vi "BonOMM-SAOMM.vi"() -> ()   [LabVIEW 2019] (continued)
                            n2356 = One Button Dialog(message="Errreur lors du déplacement de la roue") -> ()  [unwired: 1 in, 1 out]
                          }
                          frame True {
                          }
                        }
                      }
                      frame True {
                      }
                    }
                  }
                  frame #3 {
                    w6291 = u8 0 ("byte count")
                    w6301 = FALSE
                    n2357 = local read "Annulation en cours"() -> (w6288:bool)
                    n2358 = case shown="Faux" w6288 {
                      tunnel: w6300 -> [w6323 _]
                      frame False {
                        n2359 = call "MC-BonOMM_talker.vi"("MC-BonOMM VRN"=w6323, "Commande"="q" ("write buffer"), "byte count"=u32 1, "Timeout (ms)"=1000, "answer=command?"=FALSE) -> ("Answer"=w6318:string, "ok ?"=w6317:bool)
                        n2360 = local write "MC_connect"(w6317) -> ()
                        n2361 = Decimal String To Number(string=w6318) -> (number=w6322:i32)  [unwired: 2 in, 1 out]
                        n2362 = local write "F#"(w6322) -> ()
                        n2363 = case shown="1..6" w6322 {
                          selector: w6322 -> [w6333 _]
                          frame 1..6 {
                            w6324 = TRUE ("enabled")
                            n2364 = Decrement(x=w6333) -> (x-1=w6325:i32)
                            n2365 = local read "Tableau des filtres"() -> (w6334:string[])
                            n2366 = Index Array(array=w6334, index=w6325) -> (element=w6326:string)
                            n2367 = Number To Decimal String(number=w6325, width (-)=i16 1) -> (decimal integer string=w6330:string)
                            n2368 = local write "filtre_nom"(w6326) -> ()
                            n2369 = Concatenate Strings("raf_", w6326, "@@", w6330) -> (w6332:string)
                            n2370 = Current VI's Menubar() -> (w6331:refnum<k9>)
                            n2371 = Set Menu Item Info(6:w6324, 7:w6332, 9:w6324, 10:w6326, 11:w6331) -> ()  [unwired: 2 in, 2 out]
                          }
                          frame 0, Default {
                            n2372 = local write "filtre_nom"("") -> ()
                          }
                        }
                      }
                      frame True {
                        n2373 = local read "MC-BonOMM VRN"() -> (w6337:refnum<visa-resource-name>)
                        n2374 = local read "Périphérique"() -> (w6341:u16)
                        n2375 = VISA Write(VISA resource name=w6337, write buffer="r") -> (VISA resource name out=w6338:refnum<visa-resource-name>)  [unwired: 1 in, 2 out]
                        n2376 = Equal To 0?(x=w6341) -> (x = 0?=w6342:bool)
                        n2377 = Select(t="f", s=w6342, f="o") -> (s? t:f=w6345:string)
                        n2378 = flat-sequence {
                          tunnel: w6338 -> [w6367]
                          tunnel: [w6367] -> w6348
                          frame #0 {
                            n2379 = Wait (ms)(milliseconds to wait=u32 2000) -> ()  [unwired: 1 out]
                          }
                        }
                        n2380 = call "MC-BonOMM_talker.vi"("MC-BonOMM VRN"=w6348, "Commande"=w6345, "byte count"=u32 1, "Timeout (ms)"=2000, "answer=command?"=TRUE) -> ("ok ?"=w6336:bool)  [unwired: 1 out]
                        n2381 = local write "MC_connect"(w6336) -> ()
                        n2382 = case shown="Vrai" w6336 {
                          tunnel: w6348 -> [_ w6350]
                          frame False {
                            n2383 = One Button Dialog(message="Erreur lors de l'arrêt, essayez \"reconnecter\"") -> ()  [unwired: 1 in, 1 out]
                          }
                          frame True {
                            n2384 = flat-sequence {
                              tunnel: [w6360] -> w6351
                              tunnel: w6350 -> [w6359]
                              frame #0 {
                                n2385 = Wait (ms)(milliseconds to wait=u32 500) -> ()  [unwired: 1 out]
                              }
                              frame #1 {
                                n2386 = call "MC-BonOMM_talker.vi"("MC-BonOMM VRN"=w6359, "Commande"="q", "byte count"=u32 1, "Timeout (ms)"=8000, "answer=command?"=FALSE) -> ("Answer"=w6355:string, "ok ?"=w6354:bool)
                                n2387 = local write "MC_connect"(w6354) -> ()
                                n2388 = Decimal String To Number(string=w6355) -> (number=w6360:i32)  [unwired: 2 in, 1 out]
                              }
                            }
                            n2389 = local write "F#"(w6351) -> ()
                            n2390 = case shown="1..6" w6351 {
                              selector: w6351 -> [w6361 _]
                              frame 1..6 {
                                n2391 = Decrement(x=w6361) -> (x-1=w6364:i32)
                                n2392 = local read "Tableau des filtres"() -> (w6362:string[])
                                n2393 = Index Array(array=w6362, index=w6364) -> (element=w6363:string)
                                n2394 = local write "filtre_nom"(w6363) -> ()
                              }
                              frame 0, Default {
                                n2395 = local write "filtre_nom"("") -> ()
                              }
                            }
                          }
                        }
                      }
                    }
                    n2396 = property on="ChoixFiltre" class="Clust (strict)"() -> ("Controls[]"=w6302:refnum<vi>[])  [unwired: 2 in, 2 out]
                    n2397 = Index Array(array=w6302, index #1=0 ("indice"), index #2=1 ("indice"), index #3=2 ("indice"), index #4=3 ("indice"), index #5=4 ("indice"), index #6=5 ("indice")) -> (element #1=w6304:refnum<vi>, element #2=w6305:refnum<vi>, element #3=w6306:refnum<vi>, element #4=w6307:refnum<vi>, element #5=w6308:refnum<vi>, element #6=w6309:refnum<vi>)
                    n2398 = property class="Cmde"(reference=w6304, "Blinking"=w6301) -> (reference out=w6299:refnum<vi>)  [unwired: 1 in, 1 out]
                    n2399 = property class="Cmde"(reference=w6305, "Blinking"=w6301) -> (reference out=w6298:refnum<vi>)  [unwired: 1 in, 1 out]
                    n2400 = property class="Cmde"(reference=w6306, "Blinking"=w6301) -> (reference out=w6297:refnum<vi>)  [unwired: 1 in, 1 out]
                    n2401 = property class="Cmde"(reference=w6307, "Blinking"=w6301) -> (reference out=w6296:refnum<vi>)  [unwired: 1 in, 1 out]
                    n2402 = property class="Cmde"(reference=w6308, "Blinking"=w6301) -> (reference out=w6295:refnum<vi>)  [unwired: 1 in, 1 out]
                    n2403 = property class="Cmde"(reference=w6309, "Blinking"=w6301) -> (reference out=w6294:refnum<vi>)  [unwired: 1 in, 1 out]
                    n2404 = Bundle(w6301, w6301, w6301, w6301, w6301, w6301) -> (w6315:cluster{bool, bool, bool, bool, bool, bool})  [unwired: 1 in]
                    n2405 = property class="Cmde"(reference=w6299, "Disabled"=w6291) -> ()  [unwired: 1 in, 2 out]
                    n2406 = property class="Cmde"(reference=w6298, "Disabled"=w6291) -> ()  [unwired: 1 in, 2 out]
                    n2407 = property class="Cmde"(reference=w6297, "Disabled"=w6291) -> ()  [unwired: 1 in, 2 out]
                    n2408 = property class="Cmde"(reference=w6296, "Disabled"=w6291) -> ()  [unwired: 1 in, 2 out]
                    n2409 = property class="Cmde"(reference=w6295, "Disabled"=w6291) -> ()  [unwired: 1 in, 2 out]
                    n2410 = local read "Périphérique"() -> (w6293:u16)
                    n2411 = property on="ChoixFiltre" class="Clust (strict)"("Value"=w6315) -> ()  [unwired: 2 in, 2 out]
                    n2412 = Equal To 0?(x=w6293) -> (x = 0?=w6292:bool)
                    n2413 = Select(t=w6291, s=w6292, f=u8 2) -> (s? t:f=w6289:u8)
                    n2414 = property class="Cmde"(reference=w6294, "Disabled"=w6289) -> ()  [unwired: 1 in, 2 out]
                  }
                }
              }
              event "Périphérique", "reconnect": Value Change {
                n2415 = event-data() -> ()  [unwired: 1 in, 5 out]
                n2416 = Equal?(x="Périphérique", y=u16 3) -> (x = y?=w6388:bool)
                n2417 = Equal?(x="Périphérique", y=u16 4) -> (x = y?=w6391:bool)
                n2418 = property on="AngOK" class="Bool"("Visible"=w6391) -> ()  [unwired: 2 in, 2 out]
                n2419 = property on="PAS" class="NumNb (strict)"("Visible"=w6391) -> ()  [unwired: 2 in, 2 out]
                n2420 = property on="ANG+" class="Bool"("Visible"=w6391) -> ()  [unwired: 2 in, 2 out]
                n2421 = property on="Set angle" class="NumNb (strict)"("Visible"=w6391) -> ()  [unwired: 2 in, 2 out]
                n2422 = property on="ANG-" class="Bool"("Visible"=w6391) -> ()  [unwired: 2 in, 2 out]
                n2423 = property on="Arc" class="Bool (strict)"("Visible"=w6388) -> ()  [unwired: 2 in, 2 out]
                n2424 = property on="Flat" class="Bool (strict)"("Visible"=w6388) -> ()  [unwired: 2 in, 2 out]
                n2425 = property on="Néon" class="Bool (strict)"("Visible"=w6388) -> ()  [unwired: 2 in, 2 out]
                n2426 = Equal?(x="Périphérique", y=u16 2) -> (x = y?=w6379:bool)
                n2427 = local write "reconnect"(FALSE ("reconnect")) -> ()
                n2428 = property on="SET ZERO" class="Bool"("Visible"=w6379) -> ()  [unwired: 2 in, 2 out]
                n2429 = property on="ST+" class="Bool (strict)"("Visible"=w6379) -> ()  [unwired: 2 in, 2 out]
                n2430 = property on="ST-" class="Bool (strict)"("Visible"=w6379) -> ()  [unwired: 2 in, 2 out]
                n2431 = property on="ST_RAZ" class="Bool"("Visible"=w6379) -> ()  [unwired: 2 in, 2 out]
                n2432 = property on="ST_SPD" class="Gliss (strict)"("Visible"=w6379) -> ()  [unwired: 2 in, 2 out]
                n2433 = Equal?(x="Périphérique", y=u16 0) -> (x = y?=w6381:bool)
                n2434 = Equal?(x="Périphérique", y=u16 1) -> (x = y?=w6380:bool)
                n2435 = Or(x=w6381, y=w6380) -> (x .or. y?=w6369:bool)
                n2436 = Select(t=u8 0 ("y"), s=w6381, f=u8 2 ("y")) -> (s? t:f=w6384:u8)
                n2437 = property on="filtre #6" class="Bool (strict)"("Disabled"=w6384) -> ()  [unwired: 2 in, 2 out]
                n2438 = Build Array(w6381, w6380, w6379) -> (w6378:bool[])
                n2439 = Or(x=w6369, y=w6379) -> (x .or. y?=w6370:bool)
                n2440 = property on="reconnect" class="Bool (strict)"("Visible"=w6370) -> ()  [unwired: 2 in, 2 out]
                n2441 = Boolean Array To Number(Boolean array=w6378) -> (number=w6377:u32)
                n2442 = property on="ChoixFiltre" class="Clust (strict)"("Visible"=w6369) -> ()  [unwired: 2 in, 2 out]
                n2443 = property on="filtre_nom" class="Ch"("Visible"=w6369) -> ()  [unwired: 2 in, 2 out]
                n2444 = property on="q-raf" class="Bool (strict)"("Visible"=w6369) -> ()  [unwired: 2 in, 2 out]
                n2445 = property on="cancel-raf" class="Bool (strict)"("Visible"=w6369) -> ()  [unwired: 2 in, 2 out]
                n2446 = property on="change_filtre_liste" class="Bool (strict)"("Visible"=w6369) -> ()  [unwired: 2 in, 2 out]
                n2447 = property on="F#" class="NumNb (strict)"("Visible"=w6369) -> ()  [unwired: 2 in, 2 out]
                n2448 = case shown="Vrai" w6370 {
                  tunnel: w6377 -> [_ w6394]
                  frame False {
                  }
                  frame True {
                    n2449 = flat-sequence {
                      tunnel: w6394 -> [w6398]
                      tunnel: [w6398] -> w6393
                      tunnel: w6393 -> [w6418]
                      frame #0 {
                        n2450 = flat-sequence {
                          tunnel: w6395 -> [w6402]
                          frame #0 {
                            n2451 = Wait (ms)(milliseconds to wait=u32 2000) -> ()  [unwired: 1 out]
                          }
                          frame #1 {
                            n2452 = property class="Instr"(reference=w6402) -> (reference out=w6401:refnum<visa-resource-name>, "Serial Settings:Number of Bytes at Serial Port"=w6400:u32)  [unwired: 1 in, 1 out]
                            n2453 = local write "MC_connect"(FALSE ("MC_connect")) -> ()
                            n2454 = VISA Read(VISA resource name=w6401, byte count=w6400) -> ()  [unwired: 1 in, 4 out]
                          }
                        }
                        n2455 = local read "MC-BonOMM VRN"() -> (w6397:refnum<visa-resource-name>)
                        n2456 = VISA Write(VISA resource name=w6397, write buffer="r" ("Commande")) -> (VISA resource name out=w6395:refnum<visa-resource-name>)  [unwired: 1 in, 2 out]
                      }
                      frame #1 {
                        n2457 = local read "MC-BonOMM VRN"() -> (w6414:refnum<visa-resource-name>)
                        n2458 = call "MC-BonOMM_talker.vi"("MC-BonOMM VRN"=w6414, "Commande"="m", "byte count"=u32 1, "Timeout (ms)"=2000, "answer=command?"=FALSE) -> ("Answer"=w6408:string, "ok ?"=w6411:bool)
                        n2459 = Equal?(x="f", y=w6408) -> (x = y?=w6407:bool)
                        n2460 = Equal?(x=w6408, y="x") -> (x = y?=w6406:bool)
                        n2461 = Or(x=w6407, y=w6406) -> (x .or. y?=w6405:bool)
                        n2462 = And(x=w6405, y=w6411) -> (x .and. y?=w6412:bool)
                        n2463 = case shown="Vrai" w6412 {
                          tunnel: w6418 -> [_ w6424]
                          tunnel: [w6419 w6423] -> w6404
                          frame False {
                            n2464 = One Button Dialog(message="Problème de communication avec MC-BonOMM", button name ("OK")="Oups :(") -> (true=w6420:bool)
                            n2465 = Not(x=w6420) -> (.not. x?=w6419:bool)
                          }
                          frame True {
                            n2466 = stacked-sequence {
                              tunnel: w6424 -> [w6429 w6455]
                              tunnel: [_ w6453] -> w6423
                              frame #0 {
                                n2467 = local read "MC-BonOMM VRN"() -> (w6431:refnum<visa-resource-name>)
                                n2468 = case shown="1, Par défaut" w6429 {
                                tunnel: ["f" "o" "x"] -> w6428
                                frame 1, Default {
                                }
                                frame 2 {
                                }
                                frame 4 {
                                }
                                }
                                n2469 = call "MC-BonOMM_talker.vi"("MC-BonOMM VRN"=w6431, "Commande"=w6428, "Timeout (ms)"=2000, "answer=command?"=TRUE) -> ("ok ?"=w6425:bool)  [unwired: 1 in, 1 out]
                                n2470 = local write "MC_connect"(w6425) -> ()
                                n2471 = Equal?(x=w6428, y="f") -> (x = y?=w6426:bool)
                                n2472 = case shown="Faux" w6425 {
                                frame False {
                                n2473 = One Button Dialog(message="Erreur lors du changement de mode ...") -> ()  [unwired: 1 in, 1 out]
                                }
                                frame True {
                                }
                                }
                                n2474 = case shown="Vrai" w6426 {
                                tunnel: w6425 -> [_ w6433]
                                frame False {
                                }
                                frame True {
                                n2475 = local read "Tableau des filtres"() -> (w6437:string[])
                                n2476 = Current VI's Menubar() -> (w6434:refnum<k9>)
                                n2477 = for {
                                tunnel: w6437 -> [w6440] mode=indexing
                                tunnel: "@@" -> [w6445]
                                tunnel: "raf_" -> [w6446]
                                tunnel: w6434 -> [w6442]
                                tunnel: w6433 -> [w6441]
                                tunnel: [w6439] -> _ mode=indexing
                                i -> [w6447]
                                n2478 = Number To Decimal String(number=w6447, width (-)=i16 1) -> (decimal integer string=w6444:string)
                                n2479 = Concatenate Strings(w6446, w6440, w6445, w6444) -> (w6443:string)
                                n2480 = Set Menu Item Info(6:FALSE ("checked"), 7:w6443, 9:w6441, 10:w6440, 11:w6442) -> (0:w6439:errorcluster)  [unwired: 2 in, 1 out]
                                }
                                }
                                }
                              }
                              frame #1 {
                                n2481 = local read "MC-BonOMM VRN"() -> (w6454:refnum<visa-resource-name>)
                                n2482 = case shown="1, 2, Par défaut" w6455 {
                                tunnel: w6454 -> [w6461 w6477]
                                tunnel: [w6459 w6476] -> w6453
                                frame 1, 2, Default {
                                n2483 = call "MC-BonOMM_talker.vi"("MC-BonOMM VRN"=w6461, "Commande"="q", "byte count"=u32 1, "Timeout (ms)"=8000, "answer=command?"=FALSE) -> ("Answer"=w6460:string, "ok ?"=w6459:bool)
                                n2484 = Decimal String To Number(string=w6460) -> (number=w6463:i32)  [unwired: 2 in, 1 out]
                                n2485 = local write "F#"(w6463) -> ()
                                n2486 = case shown="1..6" w6463 {
                                selector: w6463 -> [w6473 _]
                                frame 1..6 {
                                n2487 = local read "Tableau des filtres"() -> (w6474:string[])
                                n2488 = Decrement(x=w6473) -> (x-1=w6469:i32)
                                n2489 = Index Array(array=w6474, index=w6469) -> (element=w6464:string)
                                n2490 = Number To Decimal String(number=w6469, width (-)=i16 1) -> (decimal integer string=w6468:string)
                                n2491 = Current VI's Menubar() -> (w6467:refnum<k9>)
                                n2492 = local write "filtre_nom"(w6464) -> ()
                                n2493 = Concatenate Strings("raf_", w6464, "@@", w6468) -> (w6466:string)
                                n2494 = Set Menu Item Info(6:TRUE ("enabled"), 7:w6466, 10:w6464, 11:w6467) -> ()  [unwired: 3 in, 2 out]
                                }
                                frame 0, Default {
                                n2495 = local write "filtre_nom"("") -> ()
                                }
                                }
                                }
                                frame 4 {
                                n2496 = local read "ST_SPD"() -> (w6478:dbl)
                                n2497 = call "Change_speed.vi"("ST_SPD"=w6478, "MC-BonOMM VRN"=w6477) -> ("Connected?"=w6476:bool)
                                n2498 = case shown="Faux" w6476 {
                                frame False {
                                n2499 = property on="Périphérique" class="MDér (strict)"("Value (Signaling)"=u16 3) -> ()  [unwired: 2 in, 2 out]
                                }
                                frame True {
                                }
                                }
                                }
                                }
                              }
                            }
                          }
                        }
                        "MC_connect" <- w6404
                      }
                    }
                  }
                }
                n2500 = property on="Périphérique" class="MDér (strict)"() -> ("Ring Text.Text"=w6371:string)  [unwired: 2 in, 2 out]
                n2501 = control-ref of="TERMINAL"() -> (w6376:refnum<vi>)
                n2502 = control-ref of="Indicateur d'état"() -> (w6375:refnum<vi>)
                n2503 = Concatenate Strings("Changement du périphérique pour \"", w6371, "\"") -> (w6372:string)
                n2504 = call "TERMINAL.vi"("Indicateur Refnum"=w6375, "Terminal Refnum"=w6376, "Indicateur d'état"=w6372) -> ()
              }
              event "change_filtre_liste": Value Change {
                n2505 = event-data() -> ()  [unwired: 1 in, 6 out]
                n2506 = case shown="Vrai" "change_filtre_liste" {
                  frame False {
                  }
                  frame True {
                    n2507 = flat-sequence {
                      frame #0 {
                        n2508 = local read "Tableau des filtres"() -> (w6486:string[])
                        n2509 = Current VI's Menubar() -> (w6484:refnum<k9>)
                        n2510 = local write "change_filtre_liste"(FALSE) -> ()
                        n2511 = call "RaFMenuFixer.vi"("Tableau des filtres"=w6486, "Prefix"="raf_") -> ("Item Tags"=w6482:string[])  [unwired: 8 in, 1 out]
                        n2512 = call "ChoixFiltres.vi"("Ordre des filtres Avant"=w6486) -> ("Ordre des filtres Après"=w6488:string[])
                        n2513 = Delete Menu Items(7:w6482, 8:"main_Roue à filtres" ("menu tag"), 9:w6484) -> (0:w6481:errorcluster, 3:w6485:refnum<k9>)  [unwired: 1 in]
                        n2514 = local write "Tableau des filtres"(w6488) -> ()
                        n2515 = control-ref of="TERMINAL"() -> (w6498:refnum<vi>)
                        n2516 = control-ref of="Indicateur d'état"() -> (w6499:refnum<vi>)
                        n2517 = call "RaFMenuFixer.vi"("Tableau des filtres"=w6488, "Prefix"="raf_") -> ("Item Tags"=w6489:string[], "Item Names"=w6490:string[])  [unwired: 8 in]
                        n2518 = Insert Menu Items(5:"main_Roue à filtres" ("menu tag"), 6:w6481, 7:w6489, 8:w6490, 9:w6485) -> ()  [unwired: 1 in, 3 out]
                        n2519 = call "TERMINAL.vi"("Indicateur Refnum"=w6499, "Terminal Refnum"=w6498, "Indicateur d'état"="Modification de la liste des filtres") -> ()
                        n2520 = Array Size(array=w6488) -> (size(s)=w6493:i32)
                        n2521 = Array Subset(array=w6489, index=2, length=w6493) -> ()  [unwired: 1 out]
                        n2522 = Array Subset(array=w6490, index=2, length=w6493) -> ()  [unwired: 1 out]
                      }
                      frame #1 {
                        n2523 = property on="q-raf" class="Bool (strict)"("Val(Sgnl)"=TRUE ("Value (Signaling)")) -> ()  [unwired: 2 in, 2 out]
                      }
                    }
                  }
                }
              }
              event "q-raf": Value Change {
                n2524 = event-data() -> ()  [unwired: 1 in, 6 out]
                n2525 = case shown="Vrai" "q-raf" {
                  frame False {
                  }
                  frame True {
                    n2526 = local read "MC-BonOMM VRN"() -> (w6506:refnum<visa-resource-name>)
                    n2527 = local write "q-raf"(FALSE) -> ()
                    n2528 = VISA Write(VISA resource name=w6506, write buffer="q") -> (VISA resource name out=w6507:refnum<visa-resource-name>)  [unwired: 1 in, 2 out]
                    n2529 = VISA Read(VISA resource name=w6507, byte count=u32 1) -> (read buffer=w6509:string)  [unwired: 1 in, 3 out]
                    n2530 = control-ref of="TERMINAL"() -> (w6503:refnum<vi>)
                    n2531 = control-ref of="Indicateur d'état"() -> (w6504:refnum<vi>)
                    n2532 = Decimal String To Number(string=w6509) -> (number=w6511:i32)  [unwired: 2 in, 1 out]
                    n2533 = call "TERMINAL.vi"("Indicateur Refnum"=w6504, "Terminal Refnum"=w6503, "Indicateur d'état"="Actualisation de la position de la roue à filtre") -> ()
                    n2534 = local write "F#"(w6511) -> ()
                    n2535 = case shown="1..6" w6511 {
                      selector: w6511 -> [w6523 _]
                      frame 1..6 {
                        n2536 = Decrement(x=w6523) -> (x-1=w6512:i32)
                        n2537 = local read "Tableau des filtres"() -> (w6524:string[])
                        n2538 = Index Array(array=w6524, index=w6512) -> (element=→"filtre_nom":string)
                        n2539 = local read "Tableau des filtres"() -> (w6522:string[])
                        n2540 = Index Array(array=w6522, index=w6512) -> (element=w6514:string)
                        n2541 = Number To Decimal String(number=w6512, width (-)=i16 1) -> (decimal integer string=w6518:string)
                        n2542 = Current VI's Menubar() -> (w6517:refnum<k9>)
                        n2543 = Concatenate Strings("raf_", w6514, "@@", w6518) -> (w6516:string)
                        n2544 = Set Menu Item Info(6:TRUE ("enabled"), 7:w6516, 10:w6514, 11:w6517) -> ()  [unwired: 3 in, 2 out]
                      }
                      frame 0, Default {
                        n2545 = local write "filtre_nom"("") -> ()
                      }
                    }
                  }
                }
              }
              event "AngOK": Value Change {
                n2546 = event-data() -> ("NewVal"=w6526:bool)  [unwired: 1 in, 4 out]
                n2547 = case shown="Vrai" w6526 {
                  frame False {
                  }
                  frame True {
                    # "160000 pas/tour"
                    n2548 = Divide(x="Set angle", y=360.0) -> (x/y=w6529:dbl)
                    n2549 = Multiply(x=w6529, y=160000.0) -> (x*y=w6527:dbl)
                    n2550 = To Long Integer(number=w6527) -> ()  [unwired: 1 out]
                  }
                }
              }
              event "ANG+", "ANG-": Value Change {
                n2551 = event-data() -> ()  [unwired: 1 in, 5 out]
                n2552 = case shown="Vrai" "ANG+" {
                  tunnel: "PAS" -> [_ _]
                  frame False {
                  }
                  frame True {
                  }
                }
              }
              event "Load_obj": Value Change {
                n2553 = event-data() -> ()  [unwired: 1 in, 5 out]
                n2554 = case shown="Vrai" "Load_obj" {
                  frame False {
                  }
                  frame True {
                    n2555 = property on="Obslib" class="Tbl (strict)"() -> ("Selection Start"=w6538:T44)  [unwired: 2 in, 2 out]
                    n2556 = local read "Obslib"() -> (w6550:string[][])
                    n2557 = local write "Load_obj"(FALSE ("Charger le l'objet #1")) -> ()
                    n2558 = Unbundle(w6538) -> ("Row"=w6551:i32)  [unwired: 1 out]
                    n2559 = Index Array(array=w6550, index (row)=w6551) -> (element=w6535:string[])  [unwired: 1 in]
                    n2560 = Index Array(array=w6535, index #1=0, index #2=1, index #3=2) -> (element #1=w6547:string, element #2=w6548:string, element #3=w6549:string)
                    n2561 = Concatenate Strings("Désirez-vous charger la coordonnées : \nRA = ", w6547, "\nDEC = ", w6548, "\nEpoch = ", w6549) -> (w6542:string)
                    n2562 = Two Button Dialog(message=w6542, 1:"NON" ("F button name (\"Cancel\")"), 2:"OUI" ("T button name (\"OK\")")) -> (T button?=w6546:bool)
                    n2563 = case shown="Vrai" w6546 {
                      tunnel: w6547 -> [_ w6558]
                      tunnel: w6548 -> [_ w6557]
                      tunnel: w6549 -> [_ w6556]
                      tunnel: w6535 -> [_ w6555]
                      tunnel: w6535 -> [_ w6553]
                      frame False {
                      }
                      frame True {
                        n2564 = flat-sequence {
                          tunnel: w6558 -> [w6579]
                          tunnel: w6557 -> [w6577]
                          tunnel: w6556 -> [w6576]
                          tunnel: w6555 -> [w6594]
                          tunnel: [w6585] -> w6554
                          tunnel: w6554 -> [w6601]
                          tunnel: w6553 -> [w6602]
                          frame #0 {
                            w6578 = ", "
                            w6583 = 3600.0 ("y")
                            n2565 = call "time-str-to-time-dbl-RA.vi"("Chaîne"=w6579) -> ("TCS_coords"=w6574:dbl)
                            n2566 = call "time-str-to-time-dbl-DEC.vi"("Chaîne"=w6577) -> ("TCS_coords"=w6573:dbl)
                            n2567 = call "time-str-to-time-dbl.vi"("Chaîne"=w6576) -> ("TCS_coords"=w6572:dbl)
                            n2568 = control-ref of="TERMINAL"() -> (w6582:refnum<vi>)
                            n2569 = control-ref of="Indicateur d'état"() -> (w6581:refnum<vi>)
                            n2570 = Multiply(x=w6574, y=w6583) -> (x*y=w6570:dbl)
                            n2571 = control-ref of="TCS actif"() -> (w6563:refnum<vi>)
                            n2572 = local read "TCS VRN"() -> (w6584:refnum<visa-resource-name>)
                            n2573 = local read "LST"() -> (w6566:dbl)
                            n2574 = Multiply(x=w6573, y=w6583) -> (x*y=w6571:dbl)
                            n2575 = Concatenate Strings("Chargement de l'objet : ", w6579, w6578, w6577, w6578, w6576) -> (w6575:string)
                            n2576 = Build Array(w6574, w6573, w6572) -> (w6561:dbl[])
                            n2577 = call "Object_properties.vi"("Target RA"=w6570, "Target DEC"=w6571, "Target Epoch"=w6572, "Sideral Time"=w6566) -> ("NO RA"=w6559:string, "NO DEC"=w6560:string, "NO Epoch"=w6569:dbl, "NO HA"=w6568:dbl, "NO AM"=w6567:dbl)  [unwired: 7 in]
                            n2578 = call "TERMINAL.vi"("Indicateur Refnum"=w6581, "Terminal Refnum"=w6582, "Indicateur d'état"=w6575) -> ()
                            n2579 = call "EXCOM-CMD.vi"("VRN IN"=w6584, "Bool Refnum"=w6563, "Commande #"=6, "Args"=w6561) -> ("VRN OUT"=w6564:refnum<visa-resource-name>, "Error OUT"=w6562:errorcluster)  [unwired: 9 in, 1 out]
                            n2580 = local write "TCS Error"(w6562) -> ()
                            n2581 = local write "TCS VRN"(w6564) -> ()
                            n2582 = local write "N.O. A.D."(w6559) -> ()
                            n2583 = local write "N.O. Déc."(w6560) -> ()
                            n2584 = local write "NO epoch"(w6569) -> ()
                            n2585 = local write "NO AM"(w6567) -> ()
                            n2586 = local write "NO HA"(w6568) -> ()
                            n2587 = local write "Dec_DC"(w6560) -> ()
                            n2588 = local write "AD_DC"(w6559) -> ()
                          }
                          frame #1 {
                            n2589 = Index Array(array=w6594, index #1=5 ("index"), index #2=6 ("index")) -> (element #1=w6590:string, element #2=w6591:string)
                            n2590 = Not Equal?(x=w6591, y="") -> (x != y?=w6587:bool)
                            n2591 = Not Equal?(x="", y=w6590) -> (x != y?=w6588:bool)
                            n2592 = And(x=w6588, y=w6587) -> (x .and. y?=w6586:bool)
                            n2593 = case shown="Vrai" w6586 {
                              selector: w6586 -> [w6596 _]
                              tunnel: [w6596 w6597] -> w6585
                              frame False {
                              }
                              frame True {
                                n2594 = Two Button Dialog(message="Désirez-vous également charger\nles paramètres de guidage ?  ", 1:"NON" ("F button name (\"Cancel\")"), 2:"OUI" ("T button name (\"OK\")")) -> (T button?=w6597:bool)
                              }
                            }
                          }
                          frame #2 {
                            # "Vérifier le fonctionnement réel de cette fonction ..."
                            n2595 = case shown="Vrai" w6601 {
                              tunnel: w6602 -> [_ w6623]
                              frame False {
                              }
                              frame True {
                                w6614 = 60.0 ("x")
                                n2596 = call "Time-str-array-to-time-dbl-array.vi"("Array-str"=w6623) -> ("Array-dbl"=w6624:dbl[])
                                n2597 = Index Array(array=w6624, index #1=5, index #2=6, index #3=0 ("index"), index #4=1 ("index"), index #5=7 ("index"), index #6=8 ("index")) -> (element #1=w6627:dbl, element #2=w6625:dbl, element #3=w6626:dbl, element #4=w6604:dbl, element #5=w6620:dbl, element #6=w6619:dbl)
                                n2598 = Subtract(x=w6627, y=w6626) -> (x-y=w6615:dbl)
                                n2599 = Subtract(x=w6625, y=w6604) -> (x-y=w6616:dbl)
                                n2600 = Divide(x=w6604, y=180.0) -> (x/y=w6606:dbl)
                                n2601 = To Single Precision Float(number=w6620) -> (single precision float=w6617:sgl)
                                n2602 = To Single Precision Float(number=w6619) -> (single precision float=w6618:sgl)
                                n2603 = Multiply(x=w6614, y=w6615) -> (x*y=w6612:dbl)
                                n2604 = Multiply(x=w6614, y=w6616) -> (x*y=w6613:dbl)
                                n2605 = Multiply(x=3.141592653589793, y=w6606) -> (x*y=w6605:dbl)
                                n2606 = local write "XReference"(w6617) -> ()
                                n2607 = local write "YReference"(w6618) -> ()
                                n2608 = Multiply(x=15.0, y=w6612) -> (x*y=w6610:dbl)
                                n2609 = Cosine(x=w6605) -> (cos(x)=w6609:dbl)
                                n2610 = Multiply(x=w6609, y=w6610) -> (x*y=w6608:dbl)
                                n2611 = property on="TableXYPos" class="GraphXY (strict)"("Cursor.Cursor Position:Cursor X"=w6608, "Cursor.Cursor Position:Cursor Y"=w6613) -> ()  [unwired: 2 in, 2 out]
                              }
                            }
                          }
                        }
                      }
                    }
                  }
                }
              }
              event "Centrage": Mouse Up {
                # "2 méthode en compétition ...\nPour l'instant on utilise Vrai"
                n2612 = event-data() -> ()  [unwired: 1 in, 7 out]
                n2613 = case shown="Faux" TRUE {
                  frame True {
                    # "YOffset"
                    # "XOffset"
                    # "RefY"
                    # "RefX"
                    # "ROIWidth"
                    # "ROIHeight"
                    # "Continuer?"
                    n2614 = stacked-sequence {
                      seq-local: [_ w6644 _ _ _] -> [_ _ w6668 w6696 _]
                      seq-local: [_ w6643 _ _ _] -> [_ _ _ _ _]
                      seq-local: [_ w6642 _ _ _] -> [_ _ _ _ _]
                      seq-local: [_ w6641 _ _ _] -> [_ _ _ _ _]
                      seq-local: [_ w6640 _ _ _] -> [_ _ _ _ _]
                      seq-local: [_ w6639 _ _ _] -> [_ _ _ _ _]
                      seq-local: [_ w6638 _ _ _] -> [_ _ _ _ _]
                      frame #0 {
                        n2615 = control-ref of="TERMINAL"() -> (w6636:refnum<vi>)
                        n2616 = control-ref of="Indicateur d'état"() -> (w6635:refnum<vi>)
                        n2617 = call "TERMINAL.vi"("Indicateur Refnum"=w6635, "Terminal Refnum"=w6636, "Indicateur d'état"="Lancement de la routine de centrage" ("string")) -> ()
                      }
                      frame #1 {
                        n2618 = local read "Integrating"() -> (w6651:bool)
                        n2619 = local read "SNR"() -> (w6647:dbl)
                        n2620 = local read "Servo"() -> (w6650:bool)
                        n2621 = local read "ROIXOffset"() -> (w6639:u16)
                        n2622 = local read "ROIYOffset"() -> (w6638:u16)
                        n2623 = local read "ROIHeight"() -> (w6642:u16)
                        n2624 = local read "ROIWidth"() -> (w6643:u16)
                        n2625 = local read "XROIRef"() -> (w6641:dbl)
                        n2626 = local read "YROIRef"() -> (w6640:dbl)
                        n2627 = Greater?(x=w6647, y=5.0) -> (0:w6645:bool)
                        n2628 = Not(x=w6650) -> (.not. x?=w6649:bool)
                        n2629 = Compound Arithmetic op=AND(w6645, w6651, w6649) -> (w6648:bool)
                        n2630 = case shown="Vrai" w6648 {
                          tunnel: [FALSE w6654] -> w6644
                          frame False {
                            n2631 = One Button Dialog(message="Pour lancer la routine de centrage, assurez-vous que :\n  - la caméra fonctionne et est en acquisition\n  - une étoile est présente dans le champ (SNR>5)\n  - l'asservissement n'est pas actif") -> ()  [unwired: 1 in, 1 out]
                          }
                          frame True {
                            n2632 = Two Button Dialog(message="Désirez-vous lancer la routine de centrage ?\n(ceci déplacera les tables de translaions afin\nd'envoyer l'étoile au centre de la croisée)", 1:"Non" ("T button name (\"OK\")"), 2:"Oui" ("T button name (\"OK\")")) -> (T button?=w6654:bool)
                            n2633 = case shown="Vrai" w6654 {
                              frame False {
                              }
                              frame True {
                                # "S'assure qu'on reçoit une nouvelle image ..."
                                n2634 = local read "LastImageID"() -> (w6658:u32)
                                n2635 = while {
                                tunnel: w6658 -> [w6666]
                                tunnel: [w6663] -> _
                                i -> [w6665]
                                stop <- w6664 stop-if-true
                                n2636 = local read "LastImageID"() -> (w6667:u32)
                                n2637 = Add(x=w6666, y=u32 1) -> (x+y=w6660:u32)
                                n2638 = Greater?(x=w6667, y=w6660) -> (0:w6663:bool)
                                n2639 = Wait Until Next ms Multiple(millisecond multiple=u32 100) -> ()  [unwired: 1 out]
                                n2640 = call "Max-iteration.vi"("i max"=600, "i act"=w6665, "Valeur entrante"=w6663) -> ("break ?"=w6664:bool)
                                }
                              }
                            }
                          }
                        }
                      }
                      frame #2 {
                        n2641 = case shown="Vrai" w6668 {
                          frame False {
                          }
                          frame True {
                            n2642 = local read "GuiderAstrom"() -> (w6691:T4)
                            n2643 = local read "XCentroid"() -> (w6695:dbl)
                            n2644 = local read "YCentroid"() -> (w6694:dbl)
                            n2645 = local read "XReference"() -> (w6692:dbl)
                            n2646 = local read "YReference"() -> (w6693:dbl)
                            n2647 = local read "TableAstrom"() -> (w6686:T4)
                            n2648 = call "xy2ad.vi"("Y (px)"=w6694, "X (px)"=w6695, "Astrometry"=w6691) -> ("DEC (°)"=w6689:dbl, "RA (°)"=w6690:dbl)  [unwired: 5 in, 2 out]
                            n2649 = call "xy2ad.vi"("Y (px)"=w6693, "X (px)"=w6692, "Astrometry"=w6691) -> ("DEC (°)"=w6687:dbl, "RA (°)"=w6688:dbl)  [unwired: 5 in, 2 out]
                            n2650 = call "ad2xy.vi"("DEC"=w6689, "RA"=w6690, "Astrometry"=w6686) -> ("Y"=w6684:dbl, "X"=w6685:dbl)  [unwired: 6 in, 1 out]
                            n2651 = call "ad2xy.vi"("DEC"=w6687, "RA"=w6688, "Astrometry"=w6686) -> ("Y"=w6682:dbl, "X"=w6683:dbl)  [unwired: 6 in, 1 out]
                            n2652 = local read "Position Y"() -> (w6680:dbl)
                            n2653 = local read "Position X"() -> (w6681:dbl)
                            n2654 = formula code="cibX=tabX+(cenX-RefX);\ncibY=tabY+(cenY-RefY);"("cenX"=w6685, "tabX"=w6681, "tabY"=w6680, "cenY"=w6684, "RefX"=w6683, "RefY"=w6682) -> ("cibX"=w6679:dbl, "cibY"=w6678:dbl)
                            n2655 = local read "Position Z"() -> (w6677:dbl)
                            n2656 = local read "LimXPesto"() -> (w6670:dbl)
                            n2657 = local read "BrasPesto"() -> (w6669:bool)
                            n2658 = local read "Table VRN"() -> (w6676:refnum<visa-resource-name>)
                            n2659 = local read "Table Error"() -> (w6674:errorcluster)
                            n2660 = local write "Cible X"(w6679) -> ()
                            n2661 = local write "Cible Y"(w6678) -> ()
                            n2662 = local write "Cible Z"(w6677) -> ()
                            n2663 = control-ref of="Table actif"() -> (w6671:refnum<vi>)
                            n2664 = call "Newmark-GotoAll.vi"("Table VRN IN"=w6676, "BrasPesto"=w6669, "Bool Refnum"=w6671, "LimXPesto"=w6670, "Notify?"=FALSE, "Error IN"=w6674, "Position X"=w6679, "Position Y"=w6678, "Position Z"=w6677) -> ("Table VRN OUT"=w6675:refnum<visa-resource-name>, "Error OUT"=w6673:errorcluster)  [unwired: 5 in]
                            n2665 = local write "Table VRN"(w6675) -> ()
                            n2666 = local write "Table Error"(w6673) -> ()
                          }
                        }
                      }
                      frame #3 {
                        # "Vérifie la cohérence des résultats obtenus ..."
                        n2667 = case shown="Vrai" w6696 {
                          frame False {
                          }
                          frame True {
                            # "Au centre de la caméra ?"
                            # "Près du centre ?"
                            n2668 = local read "Position X"() -> (w6698:dbl)
                            n2669 = local read "Position Y"() -> (w6699:dbl)
                            n2670 = global read "Globals.vi" "EXIT"() -> (w6700:bool)
                            n2671 = In Range and Coerce(upper limit=500000.0, x=w6698, lower limit=450000.0 ("upper limit")) -> (In Range?=w6706:bool)  [unwired: 1 out]
                            n2672 = In Range and Coerce(upper limit=500000.0 ("lower limit"), x=w6699, lower limit=450000.0 ("upper limit")) -> (In Range?=w6707:bool)  [unwired: 1 out]
                            n2673 = local write "Indicateur d'état"("Centrage : vérification des résultats" ("Indicateur d'état")) -> ()
                            n2674 = Not(x=w6700) -> (.not. x?=w6697:bool)
                            n2675 = Compound Arithmetic op=AND(w6706, w6707, w6697) -> (w6708:bool)
                            n2676 = case shown="Vrai" w6708 {
                              frame False {
                              }
                              frame True {
                                n2677 = Two Button Dialog(message="Voulez-vous utiliser ces valeurs\ncomme valeurs de centre (x,y) ?", 1:"Non" ("F button name (\"Cancel\")"), 2:"Oui" ("T button name (\"OK\")")) -> (T button?=w6709:bool)
                                n2678 = case shown="Vrai" w6709 {
                                frame False {
                                }
                                frame True {
                                n2679 = stacked-sequence {
                                seq-local: [w6713 _] -> [_ w6719]
                                seq-local: [w6714 _] -> [_ w6720]
                                frame #0 {
                                n2680 = flat-sequence {
                                tunnel: [w6716] -> w6713
                                tunnel: [w6715] -> w6714
                                frame #0 {
                                n2681 = local read "Reference Y"() -> (w6716:dbl)
                                n2682 = local read "Reference X"() -> (w6715:dbl)
                                }
                                frame #1 {
                                n2683 = local read "Position Y"() -> (w6718:dbl)
                                n2684 = local write "Reference Y"(w6718) -> ()
                                n2685 = local read "Position X"() -> (w6717:dbl)
                                n2686 = local write "Reference X"(w6717) -> ()
                                }
                                }
                                }
                                frame #1 {
                                n2687 = Two Button Dialog(message="Voulez-vous vraiment utiliser ces \nvaleurs comme valeurs de centre (x,y) ?", 1:"Non" ("F button name (\"Cancel\")"), 2:"Oui" ("T button name (\"OK\")")) -> (T button?=w6721:bool)
                                n2688 = case shown="Faux" w6721 {
                                tunnel: w6720 -> [w6725 _]
                                tunnel: w6719 -> [w6726 _]
                                frame False {
                                n2689 = local write "Reference Y"(w6726) -> ()
                                n2690 = local write "Reference X"(w6725) -> ()
                                }
                                frame True {
                                }
                                }
                                }
                                }
                                }
                                }
                              }
                            }
                          }
                        }
                      }
                      frame #4 {
                        # "Pas certain que ce soit encore très utile ..."
                        n2691 = local write "Centrage_ready"(TRUE) -> ()
                        n2692 = global write "Globals.vi" "EXIT"(FALSE) -> ()
                        n2693 = local write "Indicateur d'état"("Centrage : fin de la routine" ("Indicateur d'état")) -> ()
                      }
                    }
                  }
                  frame False {
                    # "YOffset"
                    # "XOffset"
                    # "RefY"
                    # "RefX"
                    # "ROIWidth"
                    # "ROIHeight"
                    # "Continuer?"
                    n2694 = stacked-sequence {
                      seq-local: [_ w6739 _ _ _ _] -> [_ _ w6794 w6834 _ _]
                      seq-local: [_ w6738 _ _ _ _] -> [_ _ _ _ w6874 _]
                      seq-local: [_ w6737 _ _ _ _] -> [_ _ _ _ w6873 _]
                      seq-local: [_ w6736 _ _ _ _] -> [_ _ _ _ w6868 _]
                      seq-local: [_ w6735 _ _ _ _] -> [_ _ _ _ w6867 _]
                      seq-local: [_ w6734 _ _ _ _] -> [_ _ _ _ w6866 _]
                      seq-local: [_ w6733 _ _ _ _] -> [_ _ _ _ w6865 _]
                      frame #0 {
                        n2695 = control-ref of="TERMINAL"() -> (w6731:refnum<vi>)
                        n2696 = control-ref of="Indicateur d'état"() -> (w6730:refnum<vi>)
                        n2697 = call "TERMINAL.vi"("Indicateur Refnum"=w6730, "Terminal Refnum"=w6731, "Indicateur d'état"="Lancement de la routine de centrage" ("string")) -> ()
                      }
                      frame #1 {
                        n2698 = local read "Integrating"() -> (w6746:bool)
                        n2699 = local read "SNR"() -> (w6742:dbl)
                        n2700 = local read "Servo"() -> (w6745:bool)
                        n2701 = local read "ROIXOffset"() -> (w6734:u16)
                        n2702 = local read "ROIYOffset"() -> (w6733:u16)
                        n2703 = local read "ROIHeight"() -> (w6737:u16)
                        n2704 = local read "ROIWidth"() -> (w6738:u16)
                        n2705 = local read "XROIRef"() -> (w6736:dbl)
                        n2706 = local read "YROIRef"() -> (w6735:dbl)
                        n2707 = Greater?(x=w6742, y=5.0) -> (0:w6740:bool)
                        n2708 = Not(x=w6745) -> (.not. x?=w6744:bool)
                        n2709 = Compound Arithmetic op=AND(w6740, w6746, w6744) -> (w6743:bool)
                        n2710 = case shown="Vrai" w6743 {
                          tunnel: [FALSE w6749] -> w6739
                          frame False {
                            n2711 = One Button Dialog(message="Pour lancer la routine de centrage, assurez-vous que :\n  - la caméra fonctionne et est en acquisition\n  - une étoile est présente dans le champ (SNR>5)\n  - l'asservissement n'est pas actif") -> ()  [unwired: 1 in, 1 out]
                          }
                          frame True {
                            n2712 = Two Button Dialog(message="Désirez-vous lancer la routine de centrage ?\n(ceci déplacera les tables de translaions afin\nd'envoyer l'étoile au centre de la caméra)", 1:"Non" ("T button name (\"OK\")"), 2:"Oui" ("T button name (\"OK\")")) -> (T button?=w6750:bool)
                            n2713 = case shown="Vrai" w6750 {
                              selector: w6750 -> [w6754 _]
                              tunnel: [w6754 w6769] -> w6749
                              frame False {
                              }
                              frame True {
                                # "Remplacer par\naucune erreur\n(PrAMS)"
                                n2714 = local read "ImageHeight"() -> (w6755:u16)
                                n2715 = local read "ImageWidth"() -> (w6756:u16)
                                n2716 = control-ref of="PrAMS-ACK"() -> (w6772:refnum<vi>)
                                n2717 = local read "PrAMS VRN"() -> (w6793:refnum<visa-resource-name>)
                                n2718 = local read "PrAMS Error"() -> (w6792:errorcluster)
                                n2719 = local read "MessageType"() -> (w6778:cluster{string[], u32[]})
                                n2720 = control-ref of="PrAMS actif"() -> (w6773:refnum<vi>)
                                n2721 = local read "Signature"() -> (w6779:u32)
                                n2722 = call-poly "SAOMM-Num2littleEndian.vi"("Number"=u16 0) -> ("LiitleEndianedData"=w6775:u8[])  [unwired: 14 in]
                                n2723 = call-poly "SAOMM-Num2littleEndian.vi"("Number"=u16 0) -> ("LiitleEndianedData"=w6774:u8[])  [unwired: 14 in]
                                n2724 = call-poly "SAOMM-Num2littleEndian.vi"("Number"=w6756) -> ("LiitleEndianedData"=w6767:u8[])  [unwired: 14 in]
                                n2725 = call-poly "SAOMM-Num2littleEndian.vi"("Number"=w6755) -> ("LiitleEndianedData"=w6765:u8[])  [unwired: 14 in]
                                n2726 = To Double Precision Float(number=w6756) -> (double precision float=w6760:dbl)
                                n2727 = To Double Precision Float(number=w6755) -> (double precision float=w6758:dbl)
                                n2728 = call "SAOMM-SendSET.vi"("PRAMMS-COMM IN"=w6793, "Active Refnum"=w6773, "PrAMS-ACK"=w6772, "Signature"=w6779, "Error IN"=w6792, "MessageType"=w6778, "Active SET"="emtSetROIXOffset", "Value (little endianed byte array)"=w6775) -> ("PRAMMS-COMM OUT"=w6791:refnum<visa-resource-name>, "Error OUT"=w6788:errorcluster)  [unwired: 4 in, 2 out]
                                n2729 = expression code="x/2"(w6760) -> (w6759:dbl)
                                n2730 = expression code="x/2"(w6758) -> (w6757:dbl)
                                n2731 = call "SAOMM-SendSET.vi"("PRAMMS-COMM IN"=w6791, "Active Refnum"=w6773, "PrAMS-ACK"=w6772, "Signature"=w6779, "Error IN"=w6788, "MessageType"=w6778, "Active SET"="emtSetROIYOffset", "Value (little endianed byte array)"=w6774) -> ("PRAMMS-COMM OUT"=w6790:refnum<visa-resource-name>, "Error OUT"=w6787:errorcluster)  [unwired: 4 in, 2 out]
                                n2732 = call-poly "SAOMM-Num2littleEndian.vi"("Number"=w6759) -> ("LiitleEndianedData"=w6764:u8[])  [unwired: 14 in]
                                n2733 = call-poly "SAOMM-Num2littleEndian.vi"("Number"=w6757) -> ("LiitleEndianedData"=w6761:u8[])  [unwired: 14 in]
                                n2734 = call "SAOMM-SendSET.vi"("PRAMMS-COMM IN"=w6790, "Active Refnum"=w6773, "PrAMS-ACK"=w6772, "Signature"=w6779, "Error IN"=w6787, "MessageType"=w6778, "Active SET"="emtSetROIHeight", "Value (little endianed byte array)"=w6767) -> ("PRAMMS-COMM OUT"=w6789:refnum<visa-resource-name>, "Error OUT"=w6786:errorcluster)  [unwired: 4 in, 2 out]
                                n2735 = call "SAOMM-SendSET.vi"("PRAMMS-COMM IN"=w6789, "Active Refnum"=w6773, "PrAMS-ACK"=w6772, "Signature"=w6779, "Error IN"=w6786, "MessageType"=w6778, "Active SET"="emtSetROIWidth", "Value (little endianed byte array)"=w6765) -> ("PRAMMS-COMM OUT"=w6781:refnum<visa-resource-name>, "Error OUT"=w6780:errorcluster)  [unwired: 4 in, 2 out]
                                n2736 = call "SAOMM-SendSET.vi"("PRAMMS-COMM IN"=w6781, "Active Refnum"=w6773, "PrAMS-ACK"=w6772, "Signature"=w6779, "Error IN"=w6780, "MessageType"=w6778, "Active SET"="emtSetROIXReferencePoint", "Value (little endianed byte array)"=w6764) -> ("PRAMMS-COMM OUT"=w6782:refnum<visa-resource-name>, "Error OUT"=w6783:errorcluster)  [unwired: 4 in, 2 out]
                                n2737 = call "SAOMM-SendSET.vi"("PRAMMS-COMM IN"=w6782, "Active Refnum"=w6773, "PrAMS-ACK"=w6772, "Signature"=w6779, "Error IN"=w6783, "MessageType"=w6778, "Active SET"="emtSetROIYReferencePoint", "Value (little endianed byte array)"=w6761) -> ("Error"=w6770:bool, "Error OUT"=w6771:errorcluster)  [unwired: 4 in, 2 out]
                                n2738 = local write "PrAMS Error"(w6771) -> ()
                                n2739 = Not(x=w6770) -> (.not. x?=w6769:bool)
                              }
                            }
                          }
                        }
                      }
                      frame #2 {
                        n2740 = case shown="Vrai" w6794 {
                          frame False {
                          }
                          frame True {
                            # "S'assure qu'on reçoit une nouvelle image ..."
                            n2741 = local read "LastImageID"() -> (w6796:u32)
                            n2742 = while {
                              tunnel: w6796 -> [w6832]
                              tunnel: [w6829] -> w6795
                              i -> [w6831]
                              stop <- w6830 stop-if-true
                              n2743 = local read "LastImageID"() -> (w6833:u32)
                              n2744 = Add(x=w6832, y=u32 5) -> (x+y=w6826:u32)
                              n2745 = Greater?(x=w6833, y=w6826) -> (0:w6829:bool)
                              n2746 = Wait Until Next ms Multiple(millisecond multiple=u32 100) -> ()  [unwired: 1 out]
                              n2747 = call "Max-iteration.vi"("i max"=600, "i act"=w6831, "Valeur entrante"=w6829) -> ("break ?"=w6830:bool)
                            }
                            n2748 = case shown="Vrai" w6795 {
                              frame False {
                              }
                              frame True {
                                # "Direction à confirmer ..."
                                n2749 = local read "ImageWidth"() -> (w6803:u16)
                                n2750 = local read "ImageHeight"() -> (w6802:u16)
                                n2751 = local read "Binning"() -> (w6801:u16)
                                n2752 = To Double Precision Float(number=w6803) -> (double precision float=w6805:dbl)
                                n2753 = To Double Precision Float(number=w6802) -> (double precision float=w6804:dbl)
                                n2754 = expression code="x/2"(w6805) -> (w6799:dbl)
                                n2755 = expression code="x/2"(w6804) -> (w6800:dbl)
                                n2756 = local read "XCentroid"() -> (w6811:dbl)
                                n2757 = local read "PixScale1"() -> (w6815:dbl)
                                n2758 = local read "PixScale2"() -> (w6814:dbl)
                                n2759 = local read "YCentroid"() -> (w6812:dbl)
                                n2760 = local read "arcsec/pulse"() -> (w6806:dbl)
                                n2761 = To Double Precision Float(number=w6801) -> (double precision float=w6813:dbl)
                                n2762 = formula code="deltax=cenx-refx;\ncorrx=deltax*(pxscl1*bin)/tabscl;\ndeltay=ceny-refy;\ncorry=deltay*(pxscl2*bin)/tabscl;"("pxscl1"=w6815, "pxscl2"=w6814, "bin"=w6813, "refx"=w6799, "refy"=w6800, "cenx"=w6811, "ceny"=w6812, "tabscl"=w6806) -> ("corrx"=w6807:dbl, "corry"=w6808:dbl)  [unwired: 2 out]
                                n2763 = local read "Position X"() -> (w6810:dbl)
                                n2764 = local read "Position Y"() -> (w6809:dbl)
                                n2765 = local read "Position Z"() -> (w6818:dbl)
                                n2766 = Subtract(x=w6809, y=w6808) -> (x-y=w6817:dbl)
                                n2767 = Subtract(x=w6810, y=w6807) -> (x-y=w6816:dbl)
                                n2768 = local write "Cible X"(w6816) -> ()
                                n2769 = local write "Cible Y"(w6817) -> ()
                                n2770 = local write "Cible Z"(w6818) -> ()
                                n2771 = local read "BrasPesto"() -> (w6797:bool)
                                n2772 = local read "LimXPesto"() -> (w6798:dbl)
                                n2773 = local read "Table VRN"() -> (w6824:refnum<visa-resource-name>)
                                n2774 = local read "Table Error"() -> (w6822:errorcluster)
                                n2775 = control-ref of="Table actif"() -> (w6819:refnum<vi>)
                                n2776 = call "Newmark-GotoAll.vi"("Table VRN IN"=w6824, "BrasPesto"=w6797, "Bool Refnum"=w6819, "LimXPesto"=w6798, "Notify?"=FALSE, "Error IN"=w6822, "Position X"=w6816, "Position Y"=w6817, "Position Z"=w6818) -> ("Table VRN OUT"=w6823:refnum<visa-resource-name>, "Error OUT"=w6821:errorcluster)  [unwired: 5 in]
                                n2777 = local write "Table VRN"(w6823) -> ()
                                n2778 = local write "Table Error"(w6821) -> ()
                              }
                            }
                          }
                        }
                      }
                      frame #3 {
                        # "Vérifie la cohérence des résultats obtenus ..."
                        n2779 = case shown="Vrai" w6834 {
                          frame False {
                          }
                          frame True {
                            n2780 = local read "Position X"() -> (w6836:dbl)
                            n2781 = local read "Position Y"() -> (w6837:dbl)
                            n2782 = In Range and Coerce(upper limit=500000.0, x=w6836, lower limit=450000.0 ("upper limit")) -> (In Range?=w6844:bool)  [unwired: 1 out]
                            n2783 = In Range and Coerce(upper limit=500000.0 ("lower limit"), x=w6837, lower limit=450000.0 ("upper limit")) -> (In Range?=w6845:bool)  [unwired: 1 out]
                            n2784 = local write "Indicateur d'état"("Centrage : vérification des résultats" ("Indicateur d'état")) -> ()
                            n2785 = global read "Globals.vi" "EXIT"() -> (w6838:bool)
                            n2786 = Not(x=w6838) -> (.not. x?=w6835:bool)
                            n2787 = Compound Arithmetic op=AND(w6844, w6845, w6835) -> (w6846:bool)
                            n2788 = case shown="Vrai" w6846 {
                              frame False {
                              }
                              frame True {
                                n2789 = Two Button Dialog(message="Voulez-vous utiliser ces valeurs\ncomme valeurs de centre (x,y)", 1:"Non" ("F button name (\"Cancel\")"), 2:"Oui" ("T button name (\"OK\")")) -> (T button?=w6847:bool)
                                n2790 = case shown="Vrai" w6847 {
                                frame False {
                                }
                                frame True {
                                n2791 = stacked-sequence {
                                seq-local: [w6851 _] -> [_ w6857]
                                seq-local: [w6852 _] -> [_ w6858]
                                frame #0 {
                                n2792 = flat-sequence {
                                tunnel: [w6854] -> w6851
                                tunnel: [w6853] -> w6852
                                frame #0 {
                                n2793 = local read "Reference Y"() -> (w6854:dbl)
                                n2794 = local read "Reference X"() -> (w6853:dbl)
                                }
                                frame #1 {
                                n2795 = local read "Position Y"() -> (w6856:dbl)
                                n2796 = local write "Reference Y"(w6856) -> ()
                                n2797 = local read "Position X"() -> (w6855:dbl)
                                n2798 = local write "Reference X"(w6855) -> ()
                                }
                                }
                                }
                                frame #1 {
